vi "Single GPIO.vi"() -> ()   [LabVIEW 2020, in "CTI-Scratchpad.lvlib"]
uses:
  CTI-Scratchpad.lvlib
  CTI/GPIO Number.ctl
  CTI/GPIO Direction.ctl
  CTI/Session/Session.lvclass
  CTI/VisaComms/VisaComms.lvclass
  CTI/CTI.lvlib
panel:
  in  "GPIO":T1=2
  out "Readback":bool
  in  "Control":bool
  in  "Port":refnum<visa-resource-name>="COM3"
  in  "stop":bool
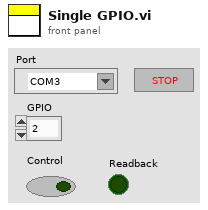
[diagram p1: front panel]
types:
  T1 = typedef "CTI.lvlib/GPIO Number.ctl" = i8
  T2 = typedef "CTI.lvlib/GPIO Direction.ctl" = enum16{"In", "Out"}
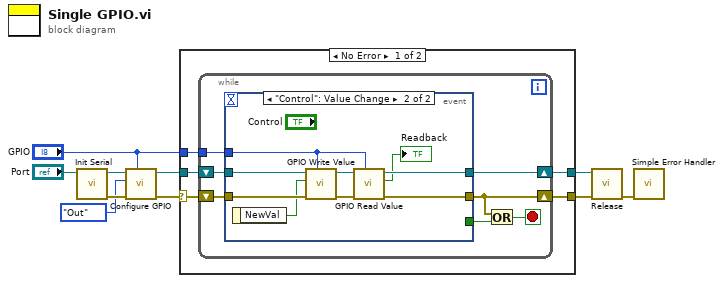
[diagram p0: block diagram]
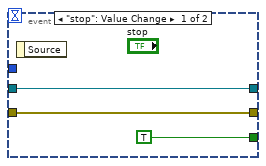
[diagram p2: hidden frame]
diagram:
  n1 = call "Init Serial.vi"("VISA resource name in"="Port") -> ("error out"=w8:errorcluster, "Session"=w9:refnum<class "Session.lvclass">)  [unwired: 8 in, 1 out]
  n2 = call "Configure GPIO.vi"("GPIO #"="GPIO", "error in (no error)"=w8, "GPIO Direction"=GPIO_Direction."Out", "Session in"=w9) -> ("error out"=w6:errorcluster, "Session out"=w7:refnum<class "Session.lvclass">)  [unwired: 6 in]
  n3 = case shown="No Error" w6 {
    selector: w6 -> [w14 w35]
    tunnel: w7 -> [w15 w36]
    tunnel: [w13 w36] -> w2
    tunnel: [w12 w35] -> w5
    tunnel: "GPIO" -> [w11 _]
    frame No Error {
      n4 = while {
        shift-right: [w20] -> w13
        shift-left: w15 -> [w22]
        shift-right: [w19] -> w12
        shift-left: w14 -> [w21]
        tunnel: w11 -> [w16]
        stop <- w18 stop-if-true
        n5 = event shown="[1] \"Control\": Value Change" {
          selector: _ -> [_ _]
          dyn-events: _ -> [_ _]
          timeout: _ -> [_ _]
          tunnel: w22 -> [w25 w34]
          tunnel: w21 -> [w24 w33]
          tunnel: [w25 w32] -> w20
          tunnel: [w24 w31] -> w19
          tunnel: [TRUE _] -> w17
          tunnel: w16 -> [_ w27]
          event "stop": Value Change {
            n6 = event-data() -> ()  [unwired: 1 in, 1 out]
          }
          event "Control": Value Change {
            n7 = event-data() -> ("NewVal"=w26:bool)  [unwired: 1 in]
            n8 = call "GPIO Write Value.vi"("GPIO #"=w27, "error in (no error)"=w33, "Value"=w26, "Session in"=w34) -> ("error out"=w29:errorcluster, "Session out"=w30:refnum<class "Session.lvclass">)  [unwired: 6 in]
            n9 = call "GPIO Read Value.vi"("GPIO #"=w27, "error in (no error)"=w29, "Session in"=w30) -> ("error out"=w31:errorcluster, "Value"=→"Readback":bool, "Session out"=w32:refnum<class "Session.lvclass">)  [unwired: 6 in]
          }
        }
        n10 = Or(x=w19, y=w17) -> (x .or. y?=w18:bool)
      }
    }
    frame Error {
    }
  }
  n11 = call-dynamic "Release.vi"("error in (no error)"=w5, "Session in"=w2) -> ("error out"=w4:errorcluster)  [unwired: 9 in]
  n12 = call <vilib>:"Simple Error Handler.vi"("error in (no error)"=w4) -> ()  [unwired: 4 in, 5 out]
